vi "dfd_FXP Quantization.vi"   [LabVIEW 2017, in "NI_DigFilter_FXP.lvlib"]
uses:
  <vilib>/addons/Digital Filter Design/NI_DigFilter_FXP.lvlib
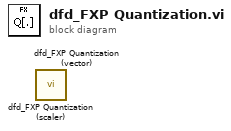
[diagram p0: block diagram]
diagram:
  n1 = call <vilib>:"dfd_FXP Quantization (scaler).vi"() -> ()  [unwired: 8 in, 1 out]
  n2 = call <vilib>:"dfd_FXP Quantization (vector).vi"() -> ()  [unwired: 8 in, 1 out]
